vi "两片74HC194的构成八位双向移位寄存器.vi"() -> ()   [LabVIEW 2018]
panel:
  in  "确定按钮":bool
  out "Q0":bool
  out "Q7":bool
  out "Q6":bool
  out "Q5":bool
  out "Q4":bool
  out "Q3":bool
  out "Q2":bool
  out "Q1":bool
  in  "D7":bool
  in  "D6":bool
  in  "D5":bool
  in  "D4":bool
  in  "D3":bool
  in  "D2":bool
  in  "D1":bool
  in  "D0":bool
  in  "DSR":bool
  in  "DSL":bool
  in  "S1":bool
  in  "S0":bool
  in  "CR0":bool
  in  "CLK":bool
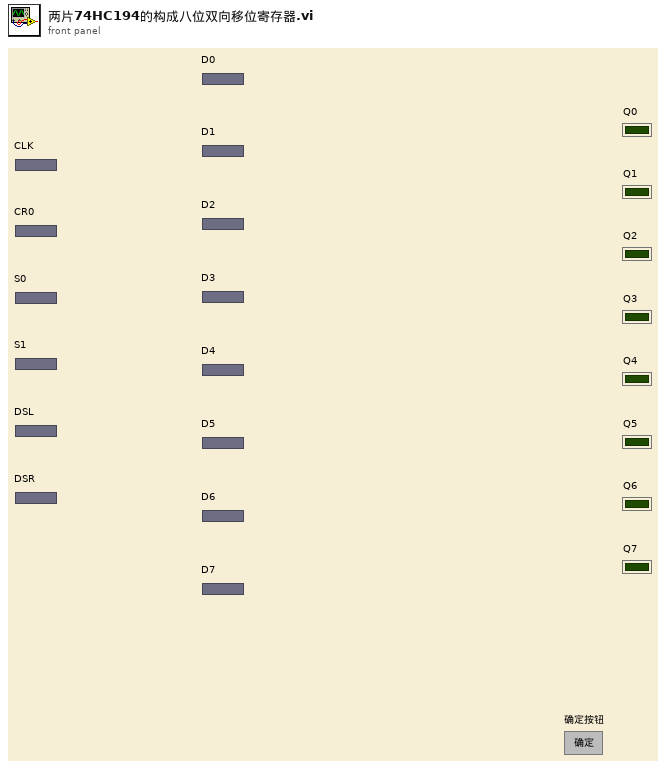
[diagram p1: front panel]
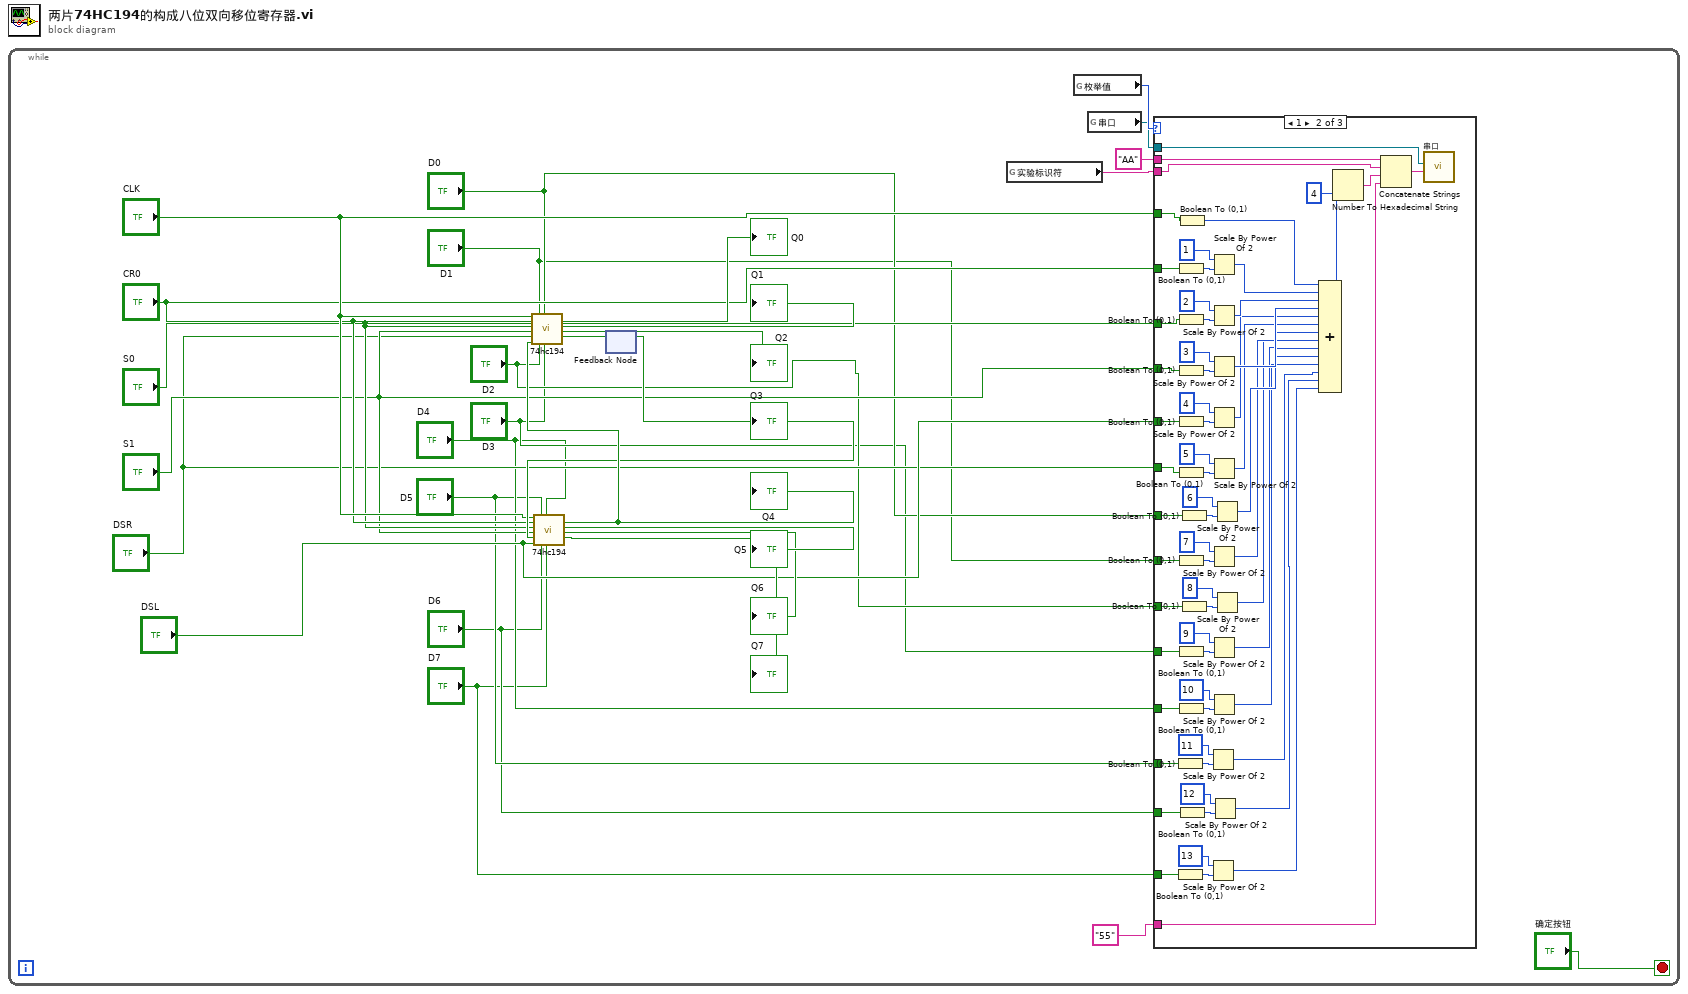
[diagram p0: block diagram]
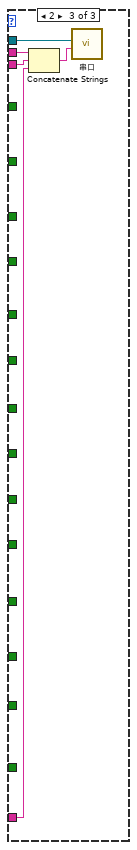
[diagram p3: hidden frame]
diagram:
  n1 = while {
    stop <- "确定按钮" stop-if-true
    n2 = feedback #1() -> (w21:bool)  [unwired: 1 in]
    "Q3" <- w21
    n3 = call "74hc194.vi"("cp"="CLK", "CR`"="CR0", "S0"="S0", "S1"="S1", "Dsr"=w21, "Dsl"="DSL", "D1"="D5", "D2"="D6", "D0"="D4", "D3"="D7") -> ("Q0"=w23:bool, "Q1"=→"Q5":bool, "Q2"=→"Q6":bool, "Q3"=→"Q7":bool)  [unwired: 6 in]
    "Q4" <- w23
    n4 = call "74hc194.vi"("cp"="CLK", "CR`"="CR0", "S0"="S0", "S1"="S1", "Dsr"="DSR", "Dsl"=w23, "D1"="D1", "D2"="D2", "D0"="D0", "D3"="D3") -> ("Q0"=→"Q0":bool, "Q1"=→"Q1":bool, "Q2"=→"Q2":bool, "Q3"=w22:bool)  [unwired: 6 in]
    n5 = feedback-in #1(w22) -> ()
    n6 = global read "全局变量.vi" "实验标识符"() -> (w17:string)
    n7 = global read "全局变量.vi" "枚举值"() -> (w19:i8)
    n8 = global read "全局变量.vi" "串口"() -> (w18:refnum<visa-resource-name>)
    n9 = case shown="1" w19 {
      tunnel: w18 -> [_ w86 w94]
      tunnel: w17 -> [_ w85 w95]
      tunnel: "55" -> [_ w84 w92]
      tunnel: "AA" -> [_ w83 w93]
      tunnel: "CLK" -> [_ w43 _]
      tunnel: "CR0" -> [_ w42 _]
      tunnel: "S0" -> [_ w41 _]
      tunnel: "S1" -> [_ w40 _]
      tunnel: "DSL" -> [_ w39 _]
      tunnel: "DSR" -> [_ w38 _]
      tunnel: "D0" -> [_ w37 _]
      tunnel: "D1" -> [_ w36 _]
      tunnel: "D2" -> [_ w35 _]
      tunnel: "D3" -> [_ w34 _]
      tunnel: "D4" -> [_ w33 _]
      tunnel: "D5" -> [_ w32 _]
      tunnel: "D6" -> [_ w31 _]
      tunnel: "D7" -> [_ w30 _]
      frame 0, Default {
      }
      frame 1 {
        n10 = Boolean To (0,1)(Boolean=w32) -> (0, 1=w52:i16)
        n11 = Boolean To (0,1)(Boolean=w30) -> (0, 1=w48:i16)
        n12 = Boolean To (0,1)(Boolean=w42) -> (0, 1=w88:i16)
        n13 = Boolean To (0,1)(Boolean=w41) -> (0, 1=w78:i16)
        n14 = Boolean To (0,1)(Boolean=w40) -> (0, 1=w76:i16)
        n15 = Boolean To (0,1)(Boolean=w39) -> (0, 1=w74:i16)
        n16 = Boolean To (0,1)(Boolean=w38) -> (0, 1=w72:i16)
        n17 = Boolean To (0,1)(Boolean=w36) -> (0, 1=w65:i16)
        n18 = Boolean To (0,1)(Boolean=w34) -> (0, 1=w61:i16)
        n19 = Boolean To (0,1)(Boolean=w33) -> (0, 1=w59:i16)
        n20 = Boolean To (0,1)(Boolean=w43) -> (0, 1=w90:i16)
        n21 = Boolean To (0,1)(Boolean=w31) -> (0, 1=w50:i16)
        n22 = Boolean To (0,1)(Boolean=w37) -> (0, 1=w67:i16)
        n23 = Boolean To (0,1)(Boolean=w35) -> (0, 1=w63:i16)
        n24 = Scale By Power Of 2(n=11, x=w52) -> (x*2^n=w46:i16)
        n25 = Scale By Power Of 2(n=13, x=w48) -> (x*2^n=w44:i16)
        n26 = Scale By Power Of 2(n=1, x=w88) -> (x*2^n=w89:i16)
        n27 = Scale By Power Of 2(n=2, x=w78) -> (x*2^n=w79:i16)
        n28 = Scale By Power Of 2(n=3, x=w76) -> (x*2^n=w70:i16)
        n29 = Scale By Power Of 2(n=4, x=w74) -> (x*2^n=w69:i16)
        n30 = Scale By Power Of 2(n=5, x=w72) -> (x*2^n=w68:i16)
        n31 = Scale By Power Of 2(n=7, x=w65) -> (x*2^n=w56:i16)
        n32 = Scale By Power Of 2(n=9, x=w61) -> (x*2^n=w54:i16)
        n33 = Scale By Power Of 2(n=10, x=w59) -> (x*2^n=w53:i16)
        n34 = Scale By Power Of 2(n=12, x=w50) -> (x*2^n=w45:i16)
        n35 = Scale By Power Of 2(n=6, x=w67) -> (x*2^n=w57:i16)
        n36 = Scale By Power Of 2(n=8, x=w63) -> (x*2^n=w55:i16)
        n37 = Compound Arithmetic op=ADD ("复合运算")(w90, w89, w79, w70, w69, w68, w57, w56, w55, w54, w53, w46, w45, w44) -> (w82:i16)
        n38 = Number To Hexadecimal String(1:4, 2:w82) -> (0:w80:string)
        n39 = Concatenate Strings(w83, w85, w80, w84) -> (w91:string)
        n40 = call "串口.vi"("字符串"=w91, "VISA resource name"=w86) -> ()  [unwired: 10 in]
      }
      frame 2 {
        n41 = Concatenate Strings(w93, w95, w92) -> (w96:string)
        n42 = call "串口.vi"("字符串"=w96, "VISA resource name"=w94) -> ()  [unwired: 10 in]
      }
    }
  }
